vi "Binary Block Save.vi"(0 "Data Array":dbl[](array[numeric]), 1 "file path (use dialog)":path, 5 "Number of Channels":u32, 7 "Block Size":u32, 9 "Counter In":i32, 11 "error in":errorcluster) -> (10 "Counter Out":i32, 15 "error out":errorcluster)   [LabVIEW 2015]
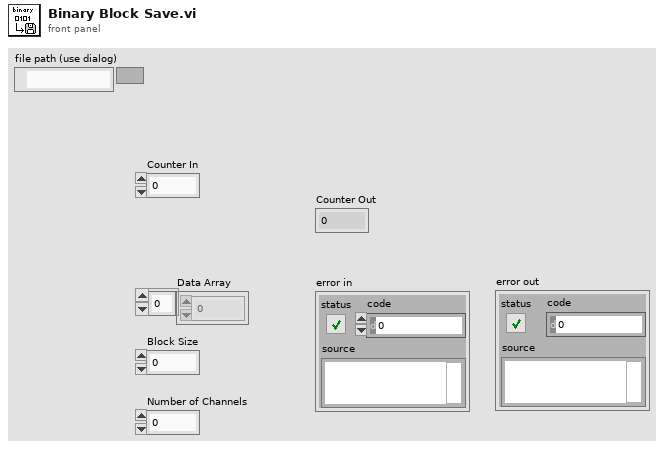
[diagram p1: front panel]
types:
  T1 = enum16{"open", "replace", "create", "open or create", "replace or create", "replace or create with confirmation"}
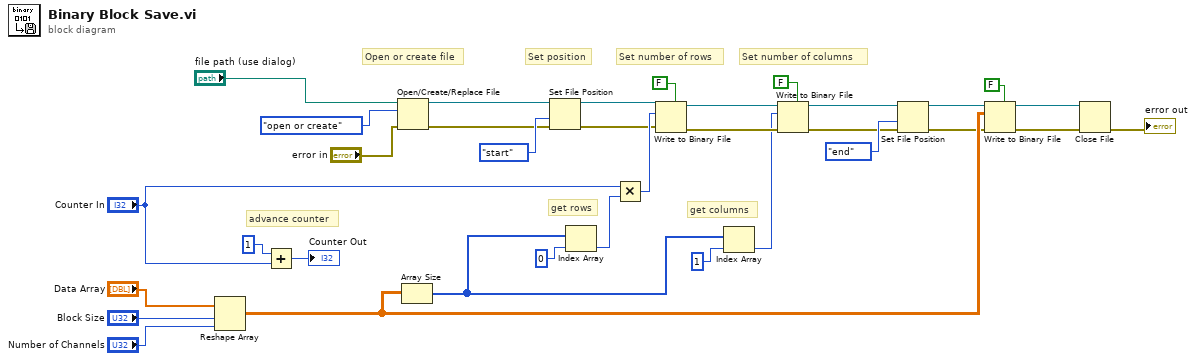
[diagram p0: block diagram]
diagram:
  # "advance counter"
  # "Set number of columns"
  # "Set number of rows"
  # "get columns"
  # "get rows"
  # "Set position"
  # "Open or create file"
  n1 = Reshape Array("Data Array", "Block Size", "Number of Channels") -> (w27:dbl[][])
  n2 = Add(x=1, y="Counter In") -> (x+y=→"Counter Out":i32)
  n3 = Open/Create/Replace File(file path (use dialog)="file path (use dialog)", error in="error in", operation (0:open)=T1."open or create") -> (refnum out=w13:refnum<file>, error out=w14:errorcluster)  [unwired: 3 in, 1 out]
  n4 = Array Size(array=w27) -> (size(s)=w20:i32[])
  n5 = Set File Position(refnum=w13, from (0:start)=enum16{"start", "end", "current"}."start", error in=w14) -> (refnum out=w24:refnum<file>, error out=w23:errorcluster)  [unwired: 1 in]
  n6 = Index Array(array=w20, index=0) -> (element=w5:i32)
  n7 = Multiply(x="Counter In", y=w5) -> (x*y=w30:i32)
  n8 = Write to Binary File(file (use dialog)=w24, data=w30, error in=w23, 5:FALSE ("prepend array or string size? (T)")) -> (refnum out=w29:refnum<file>, error out=w26:errorcluster)  [unwired: 2 in, 1 out]
  n9 = Index Array(array=w20, index=1) -> (element=w25:i32)
  n10 = Write to Binary File(file (use dialog)=w29, data=w25, error in=w26, 5:FALSE ("prepend array or string size? (T)")) -> (refnum out=w28:refnum<file>, error out=w4:errorcluster)  [unwired: 2 in, 1 out]
  n11 = Set File Position(refnum=w28, from (0:start)=enum16{"start", "end", "current"}."end", error in=w4) -> (refnum out=w31:refnum<file>, error out=w3:errorcluster)  [unwired: 1 in]
  n12 = Write to Binary File(file (use dialog)=w31, data=w27, error in=w3, 5:FALSE ("prepend array or string size? (T)")) -> (refnum out=w10:refnum<file>, error out=w9:errorcluster)  [unwired: 2 in, 1 out]
  n13 = Close File(refnum=w10, error in=w9) -> (error out=→"error out":errorcluster)  [unwired: 1 out]
